vi "configDAQ.vi"(8 "error in (no error)":errorcluster, 11 "DAQ in":refnum<class "DAQ.lvclass">) -> (0 "error out":errorcluster, 3 "DAQ out":refnum<class "DAQ.lvclass">)   [LabVIEW 2019, in "DAQ.lvclass"]
uses:
  DAQ.lvclass
  DAQ.lvclass/DAQ.ctl
  <vilib>/DAQmx/create/channels.llb/DAQmx Create Channel (AI-Voltage-Basic).vi
  <vilib>/DAQmx/configure/timing.llb/DAQmx Timing (Sample Clock).vi
panel:
  out "DAQ ref":refnum<k21>
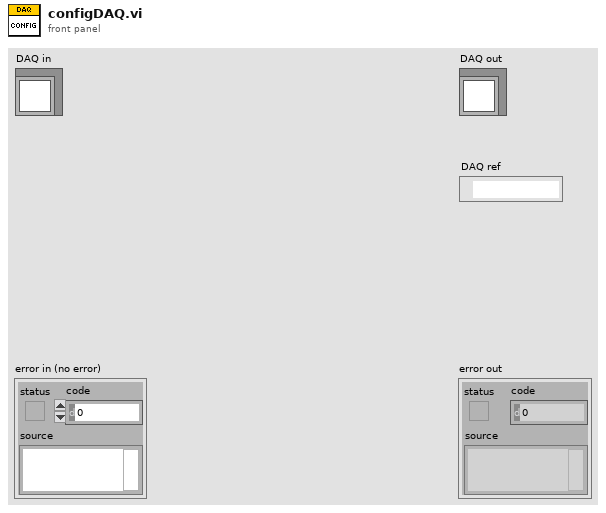
[diagram p1: front panel]
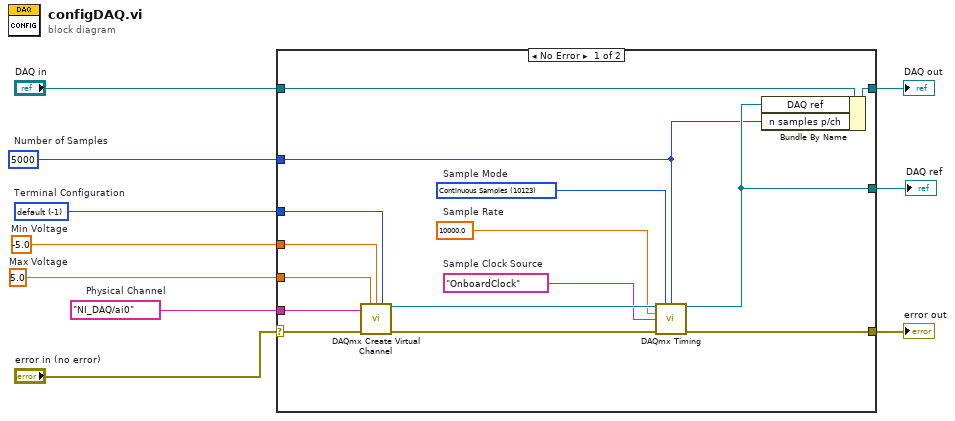
[diagram p0: block diagram]
diagram:
  w8 = tag "NI_DAQ/ai0"  # Physical Channel
  w5 = 5.0  # Max Voltage
  w6 = -5.0  # Min Voltage
  w7 = -1 items=["default"=-1, "RSE"=10083, "NRSE"=10078, "Differential"=10106, "Pseudodifferential"=12529]  # Terminal Configuration
  w1 = 5000  # Number of Samples
  n1 = case shown="No Error" "error in (no error)" {
    selector: "error in (no error)" -> [w12 w27]
    tunnel: [w25 w27] -> w10
    tunnel: "DAQ in" -> [w24 w26]
    tunnel: w8 -> [w20 _]
    tunnel: w7 -> [w19 _]
    tunnel: w6 -> [w16 _]
    tunnel: w5 -> [w15 _]
    tunnel: w1 -> [w11 _]
    tunnel: [w14 w26] -> w4
    tunnel: [w13 _] -> w3
    frame No Error {
      w18 = tag "OnboardClock"  # Sample Clock Source
      w17 = 10000.0  # Sample Rate
      w23 = 10123 items=["Finite Samples"=10178, "Continuous Samples"=10123, "Hardware Timed Single Point"=12522]  # Sample Mode
      n2 = call-poly <vilib>:"DAQmx Create Virtual Channel.vi"("maximum value"=w15, "minimum value"=w16, "input terminal configuration"=w19, "physical channels"=w20, "error in"=w12) -> ("task out"=w21:refnum<k21>, "error out"=w22:errorcluster)  [unwired: 9 in]
      n3 = call-poly <vilib>:"DAQmx Timing.vi"("task/channels in"=w21, "sample mode"=w23, "samples per channel"=w11, "rate"=w17, "source"=w18, "error in"=w22) -> ("task out"=w13:refnum<k21>, "error out"=w25:errorcluster)  [unwired: 8 in]
      n4 = Bundle By Name(cluster=w24, "DAQ ref"=w13, "n samples p/ch"=w11) -> (w14:refnum<class "DAQ.lvclass">)
    }
    frame Error {
    }
  }
  "error out" <- w10
  "DAQ out" <- w4
  "DAQ ref" <- w3
